vi "Global_ACT_Data Out.vi"() -> ()   [LabVIEW 2023, in "Angler_ACT.lvlib"]
uses:
  Angler_ACT.lvlib
panel:
  in  "ACT_Angler_Current Position":i32
  in  "ACT_Angler_Target Position":dbl
  in  "ACT_Angler_CycleTime(S)":dbl
  in  "ACT_Angler_Current Angle":dbl
  # "The Names of the Data items in the Global Variable MUST describe who the Single Writer is\nFor Actuator Globals the the naming convention is\n   \nACT_Lib Name_Data Name\n\nExamples:\nACT_Drive_X axis\nACT_Hopper_AgitatorSpeed"
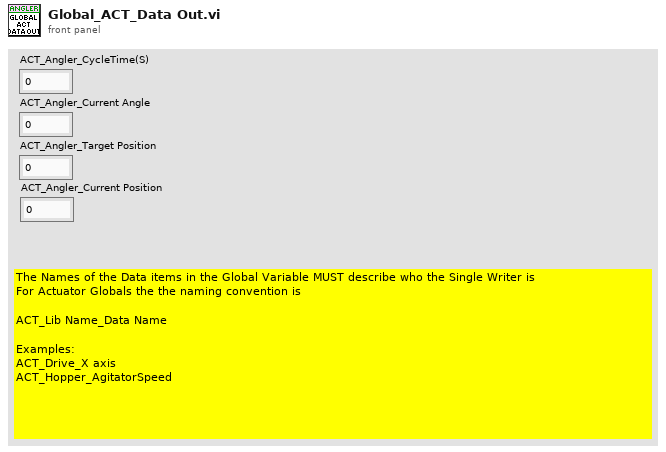
[diagram p1: front panel]
diagram:
